vi "Create.vi"(8 "Error In":errorcluster, 11 "Reader":refnum<class "Abstract.lvclass">) -> (0 "Error Out":errorcluster, 3 "Compiler":refnum<class "Compiler.lvclass">)   [LabVIEW 2018, in "Toolkit.lvlib" / "Compiler.lvclass"]
uses:
  Compiler.lvclass
  Readers/Abstract/Abstract.lvclass
  Compiler.lvclass/Compiler.ctl
  Parser/Parser.lvclass
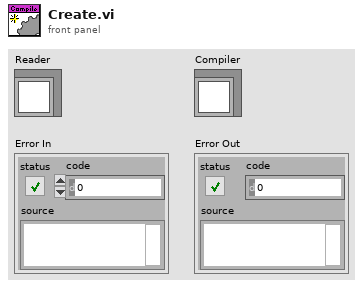
[diagram p1: front panel]
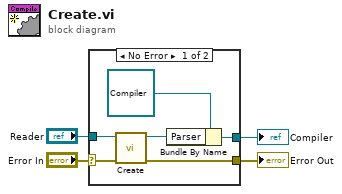
[diagram p0: block diagram]
diagram:
  n1 = case shown="No Error" "Error In" {
    selector: "Error In" -> [w10 w11]
    tunnel: [w9 w11] -> w3
    tunnel: [w6 _] -> w2
    tunnel: "Reader" -> [w8 _]
    frame No Error {
      n2 = call "Create.vi"("Error In"=w10, "Reader"=w8) -> ("Error Out"=w9:errorcluster, "Parser"=w5:refnum<class "Parser.lvclass">)  [unwired: 8 in]
      n3 = Bundle By Name(cluster=refnum<class "Compiler.lvclass"> refnum ("Mustache.lvlib:Compiler.lvclass"), "Parser"=w5) -> (w6:refnum<class "Compiler.lvclass">)
    }
    frame Error {
    }
  }
  "Error Out" <- w3
  "Compiler" <- w2
